vi "FRCts20_EspEngine_Universe.vi"(8 "error in (no error)":errorcluster, 10 "Universe":T1, 11 "httpRequestID":u32) -> (0 "error out":errorcluster, 3 "httpRequestID out":u32)   [LabVIEW 2014, in "FRCts20_EspEngine.lvlib"]
uses:
  FRCts20_EspEngine.lvlib
  TypeDefs/FRCts20_EspEngine_Universe.ctl
  TypeDefs/FRCts20_EspEngine_Team.ctl
  Web Methods/source/VI Source/Web Method Public Interface/FRCts20_WebMethods_ctl_singleTeam.ctl
  Web Methods/source/VI Source/Web Method Public Interface/FRCts20_WebMethods_ctl_teamIdentifier.ctl
  Backend/source/VI Source/FRCts20_Backend_API/FRCts20_Backend_API_SW.ctl
  Web Methods/source/VI Source/Web Method Public Interface/FRCts20_WebMethods_ctl_request.ctl
  Backend/source/VI Source/FRCts20_Backend_API/FRCts20_Backend_API_Status.ctl
  TypeDefs/FRCts20_EspEngine_Event.ctl
  Web Methods/source/VI Source/Web Method Public Interface/FRCts20_WebMethods_ctl_singleEvent.ctl
  <vilib>/wsapi/subVIs/Set Integer ESP Variable.vi
  FRCts20_EspEngine_FormatArrayOfKeysInts.vi
  FRCts20_EspEngine_FormatArrayOfKeysStrings.vi
  <vilib>/wsapi/subVIs/Set Boolean ESP Variable.vi
  <vilib>/wsapi/NI_WebServices.lvlib
  Web Methods/source/VI Source/FRCts20_WebMethods.lvlib
  Backend/source/VI Source/FRCts20_Backend_API/FRCts20_Backend_API.lvlib
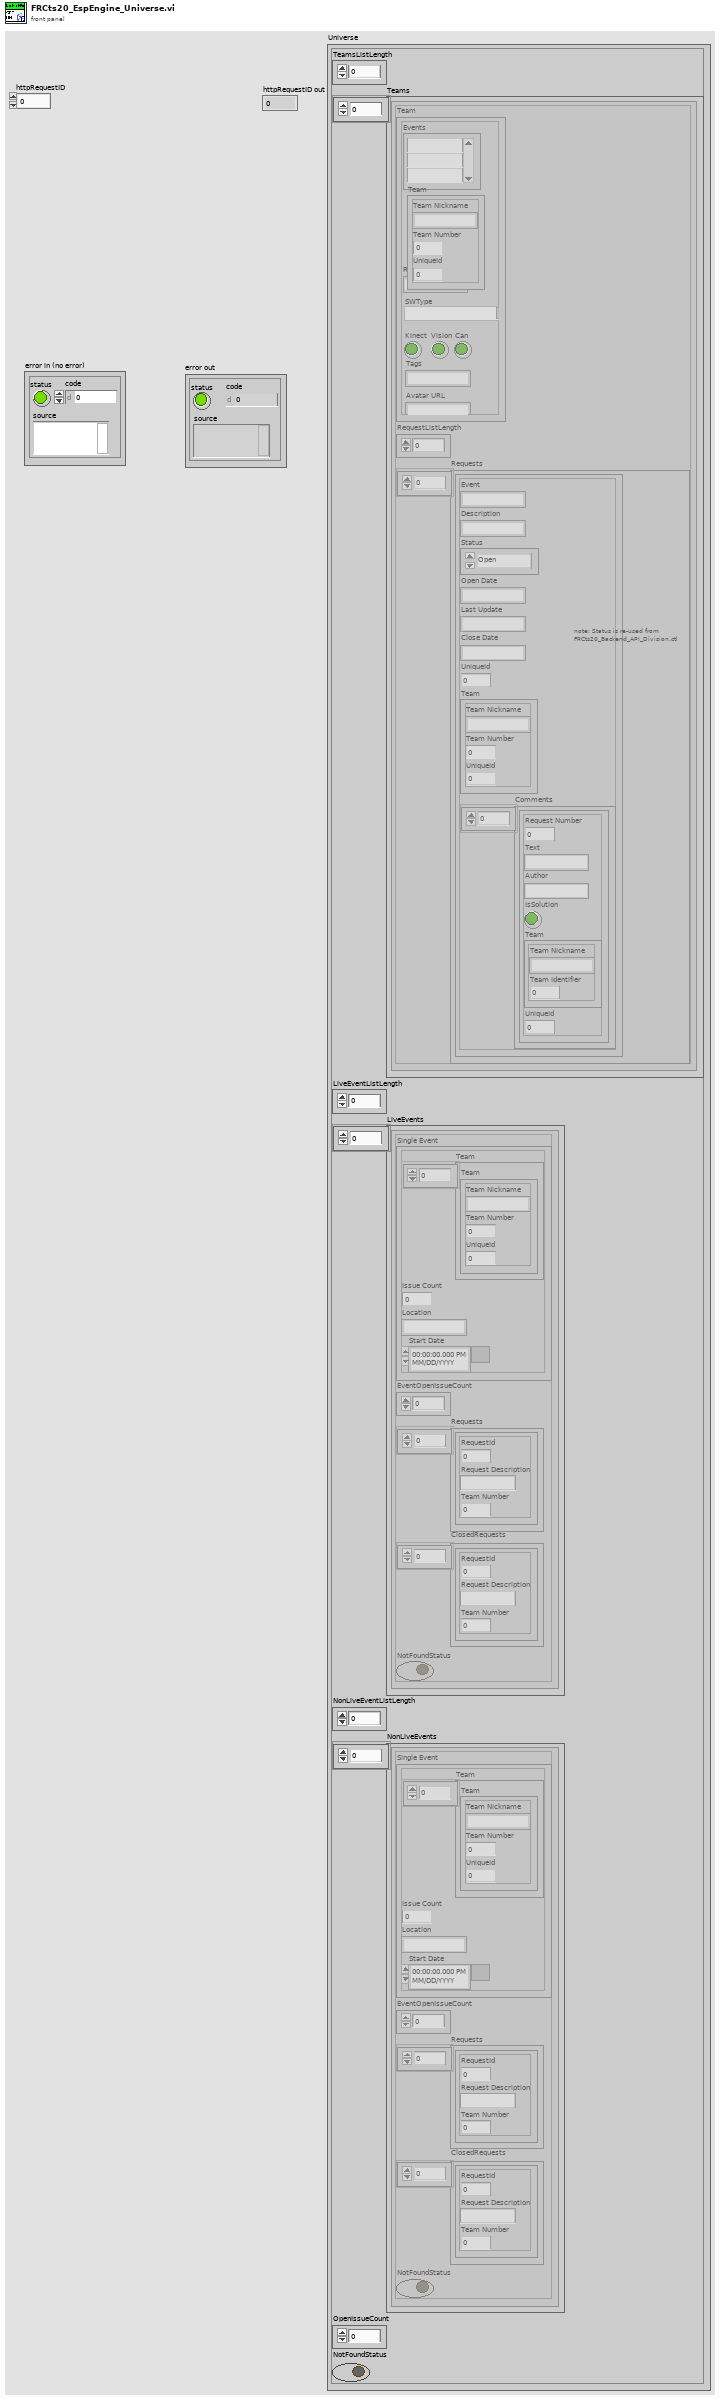
[diagram p1: front panel]
types:
  T1 = typedef "FRCts20_EspEngine.lvlib/FRCts20_EspEngine_Universe.ctl" = cluster{"TeamsListLength":i16, "Teams":T2[], "LiveEventListLength":i16, "LiveEvents":T8[], "NonLiveEventListLength":i16, "NonLiveEvents":T8[], "OpenIssueCount":i16, "NotFoundStatus":bool}
  T2 = typedef "FRCts20_EspEngine.lvlib/FRCts20_EspEngine_Team.ctl" = cluster{"Team":T3, "RequestListLength":i16, "Requests":T6[]}
  T3 = typedef "FRCts20_WebMethods.lvlib/FRCts20_WebMethods_ctl_singleTeam.ctl" = cluster{"Events":string[], "Robot Name":string, "Kinect":bool, "Vision":bool, "Can":bool, "Tags":string, "Avatar URL":string, "Team":T4, "SWType":T5}
  T4 = typedef "FRCts20_WebMethods.lvlib/FRCts20_WebMethods_ctl_teamIdentifier.ctl" = cluster{"Team Nickname":string, "Team Number ":u32, "UniqueId":u32}
  T5 = typedef "FRCts20_Backend_API.lvlib/FRCts20_Backend_API_SW.ctl" = string
  T6 = typedef "FRCts20_WebMethods.lvlib/FRCts20_WebMethods_ctl_request.ctl" = cluster{"Event":string, "Description":string, "Status":T7, "Open Date":string, "Last Update":string, "Close Date":string, "UniqueId":i32, "Team":cluster{"Team Nickname":string, "Team Number ":i32, "UniqueId":i32}, "Comments":cluster{"Request Number":dbl, "Text":string, "Author":string, "IsSolution":bool, "Team":cluster{"Team Nickname":string, "Team Identifier ":dbl}, "UniqueId":i32}[]}
  T7 = typedef "FRCts20_Backend_API.lvlib/FRCts20_Backend_API_Status.ctl" = enum16{"Open", "In Work", "Closed"}
  T8 = typedef "FRCts20_EspEngine.lvlib/FRCts20_EspEngine_Event.ctl" = cluster{"Single Event":T9, "EventOpenIssueCount":i16, "Requests":cluster{"RequestId":i32, "Request Description":string, "Team Number":i32}[], "ClosedRequests":cluster{"RequestId":i32, "Request Description":string, "Team Number":i32}[], "NotFoundStatus":bool}
  T9 = typedef "FRCts20_WebMethods.lvlib/FRCts20_WebMethods_ctl_singleEvent.ctl" = cluster{"Team":T4[], "Issue Count":i32, "Location":string, "Start Date ":timestamp}
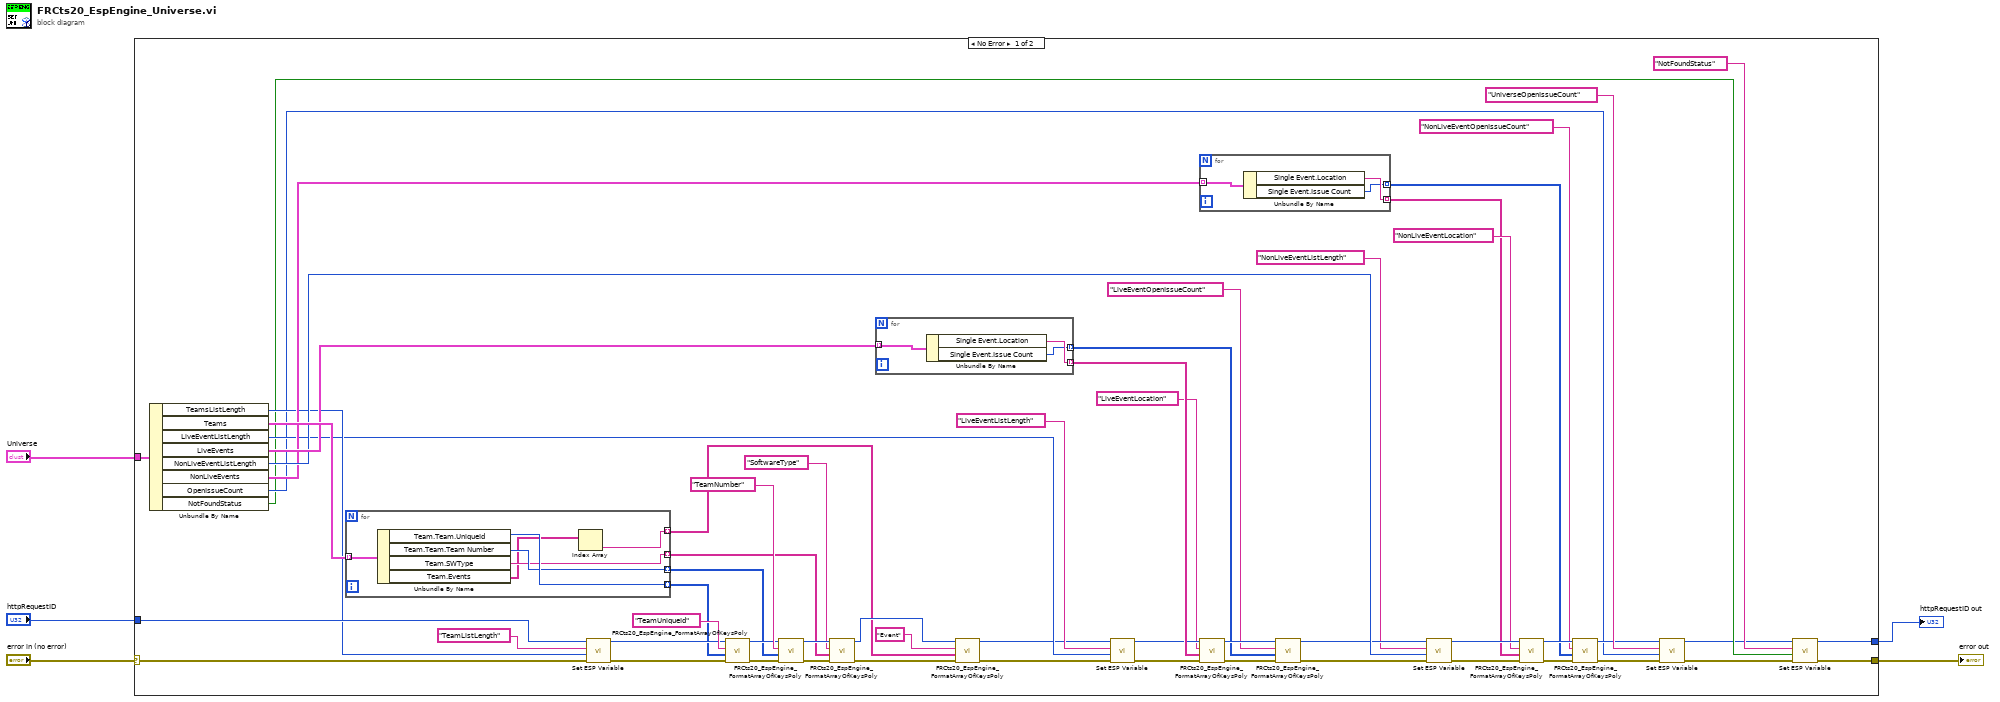
[diagram p0: block diagram]
diagram:
  n1 = case shown="No Error" "error in (no error)" {
    selector: "error in (no error)" -> [w60 w76]
    tunnel: [w8 w76] -> w5
    tunnel: "Universe" -> [w63 _]
    tunnel: "httpRequestID" -> [w62 _]
    tunnel: [w6 _] -> w1
    frame No Error {
      n2 = Unbundle By Name(w63) -> ("TeamsListLength"=w32:i16, "Teams"=w58:T2[], "LiveEventListLength"=w31:i16, "LiveEvents"=w54:T8[], "NonLiveEventListLength"=w44:i16, "NonLiveEvents"=w41:T8[], "OpenIssueCount"=w27:i16, "NotFoundStatus"=w10:bool)
      n3 = for {
        tunnel: w58 -> [w75] mode=indexing
        tunnel: [w74] -> w26 mode=indexing
        tunnel: [w73] -> w14 mode=indexing
        tunnel: [w72] -> w13 mode=indexing
        tunnel: [w70] -> w12 mode=indexing
        n4 = Unbundle By Name(w75) -> ("Team.Team.UniqueId"=w74:u32, "Team.Team.Team Number"=w73:u32, "Team.SWType"=w72:T5, "Team.Events"=w71:string[])
        n5 = Index Array(array=w71) -> (element=w70:string)  [unwired: 1 in]
      }
      n6 = call-poly <vilib>:"Set ESP Variable.vi"("error in (no error)"=w60, "value"=w32, "key"="TeamListLength", "httpRequestID"=w62) -> ("error out"=w56:errorcluster, "httpRequestID out"=w55:u32)  [unwired: 6 in]
      n7 = call-poly "FRCts20_EspEngine_FormatArrayOfKeysPoly.vi"("error IO"=w56, "Values"=w26, "KeyBaseName"="TeamUniqueId", "httpRequestID"=w55) -> ("error IO"=w18:errorcluster, "httpRequestID out"=w16:u32)  [unwired: 6 in]
      n8 = call-poly "FRCts20_EspEngine_FormatArrayOfKeysPoly.vi"("error IO"=w18, "Values"=w14, "KeyBaseName"="TeamNumber", "httpRequestID"=w16) -> ("error IO"=w25:errorcluster, "httpRequestID out"=w24:u32)  [unwired: 6 in]
      n9 = call-poly "FRCts20_EspEngine_FormatArrayOfKeysPoly.vi"("error IO"=w25, "Values"=w13, "KeyBaseName"="SoftwareType", "httpRequestID"=w24) -> ("error IO"=w22:errorcluster, "httpRequestID out"=w23:u32)  [unwired: 6 in]
      n10 = for {
        tunnel: w54 -> [w69] mode=indexing
        tunnel: [w68] -> w53 mode=indexing
        tunnel: [w67] -> w47 mode=indexing
        n11 = Unbundle By Name(w69) -> ("Single Event.Location"=w68:string, "Single Event.Issue Count"=w67:i32)
      }
      n12 = call-poly "FRCts20_EspEngine_FormatArrayOfKeysPoly.vi"("error IO"=w22, "Values"=w12, "KeyBaseName"="Event", "httpRequestID"=w23) -> ("error IO"=w17:errorcluster, "httpRequestID out"=w15:u32)  [unwired: 6 in]
      n13 = call-poly <vilib>:"Set ESP Variable.vi"("error in (no error)"=w17, "value"=w31, "key"="LiveEventListLength", "httpRequestID"=w15) -> ("error out"=w52:errorcluster, "httpRequestID out"=w51:u32)  [unwired: 6 in]
      n14 = for {
        tunnel: w41 -> [w66] mode=indexing
        tunnel: [w65] -> w35 mode=indexing
        tunnel: [w64] -> w33 mode=indexing
        n15 = Unbundle By Name(w66) -> ("Single Event.Location"=w65:string, "Single Event.Issue Count"=w64:i32)
      }
      n16 = call-poly "FRCts20_EspEngine_FormatArrayOfKeysPoly.vi"("error IO"=w52, "Values"=w53, "KeyBaseName"="LiveEventLocation", "httpRequestID"=w51) -> ("error IO"=w49:errorcluster, "httpRequestID out"=w48:u32)  [unwired: 6 in]
      n17 = call-poly "FRCts20_EspEngine_FormatArrayOfKeysPoly.vi"("error IO"=w49, "Values"=w47, "KeyBaseName"="LiveEventOpenIssueCount", "httpRequestID"=w48) -> ("error IO"=w45:errorcluster, "httpRequestID out"=w43:u32)  [unwired: 6 in]
      n18 = call-poly <vilib>:"Set ESP Variable.vi"("error in (no error)"=w45, "value"=w44, "key"="NonLiveEventListLength", "httpRequestID"=w43) -> ("error out"=w40:errorcluster, "httpRequestID out"=w38:u32)  [unwired: 6 in]
      n19 = call-poly "FRCts20_EspEngine_FormatArrayOfKeysPoly.vi"("error IO"=w40, "Values"=w35, "KeyBaseName"="NonLiveEventLocation", "httpRequestID"=w38) -> ("error IO"=w39:errorcluster, "httpRequestID out"=w37:u32)  [unwired: 6 in]
      n20 = call-poly "FRCts20_EspEngine_FormatArrayOfKeysPoly.vi"("error IO"=w39, "Values"=w33, "KeyBaseName"="NonLiveEventOpenIssueCount", "httpRequestID"=w37) -> ("error IO"=w29:errorcluster, "httpRequestID out"=w28:u32)  [unwired: 6 in]
      n21 = call-poly <vilib>:"Set ESP Variable.vi"("error in (no error)"=w29, "value"=w27, "key"="UniverseOpenIssueCount", "httpRequestID"=w28) -> ("error out"=w9:errorcluster, "httpRequestID out"=w7:u32)  [unwired: 6 in]
      n22 = call-poly <vilib>:"Set ESP Variable.vi"("error in (no error)"=w9, "value"=w10, "key"="NotFoundStatus", "httpRequestID"=w7) -> ("error out"=w8:errorcluster, "httpRequestID out"=w6:u32)  [unwired: 6 in]
    }
    frame Error {
    }
  }
  "error out" <- w5
  "httpRequestID out" <- w1
